vi "formatMsgDetails.vi"(8 "error in (no error)":errorcluster, 10 "msgCluster":T1={"msgName"="move", "msgDetails"=""}, 11 "TcpServerBase in":refnum<class "TcpServerBase.lvclass">) -> (0 "error out":errorcluster, 2 "jsonString":string, 3 "TcpServerBase out":refnum<class "TcpServerBase.lvclass">)   [LabVIEW 2018, in "TcpServerBase.lvclass"]
doc: "Convert the event or the telemetry message into a JSON format. If the message name has an empty string, an error will be created to inform other processes about this error."
uses:
  TcpServerBase.lvclass
  typedef/msgTypeDef.ctl
  <vilib>/Utility/error.llb/Error Cluster From Error Code.vi
  <vilib>/ErrorRing/Error Ring.xnode
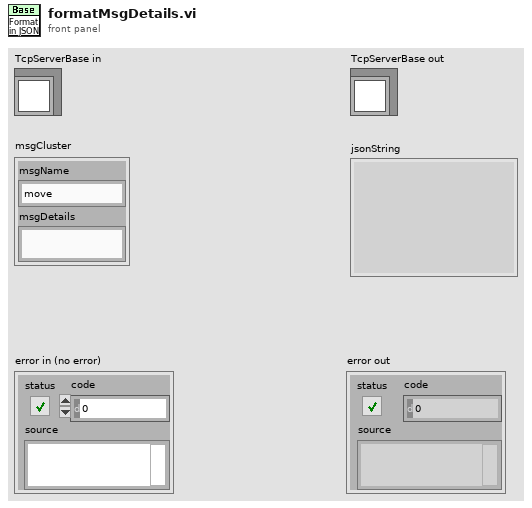
[diagram p1: front panel]
types:
  T1 = typedef "TcpServerBase.lvclass/msgTypeDef.ctl" = cluster{"msgName":string, "msgDetails":string}
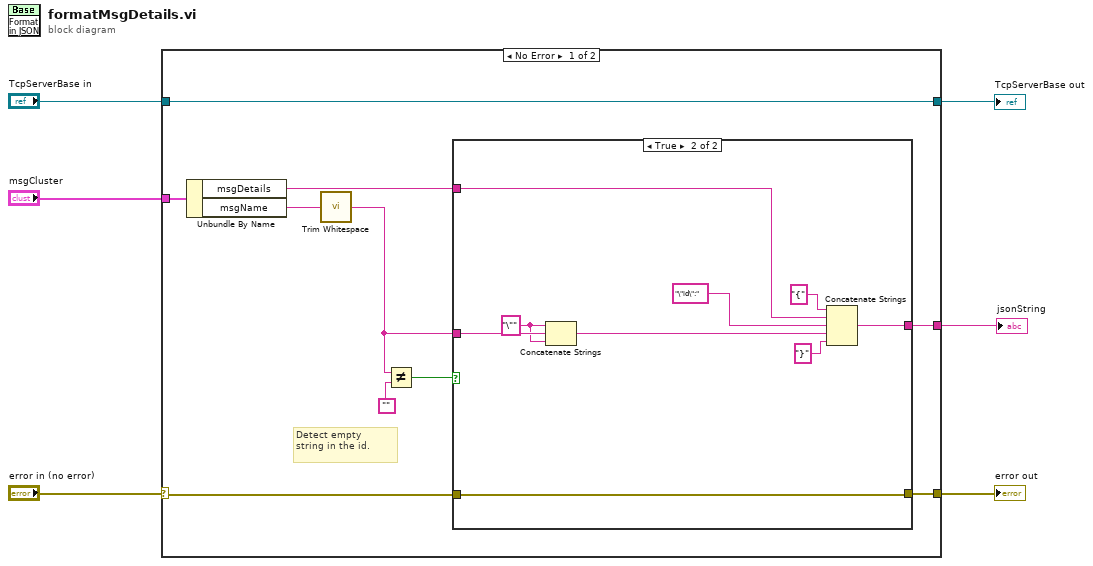
[diagram p0: block diagram]
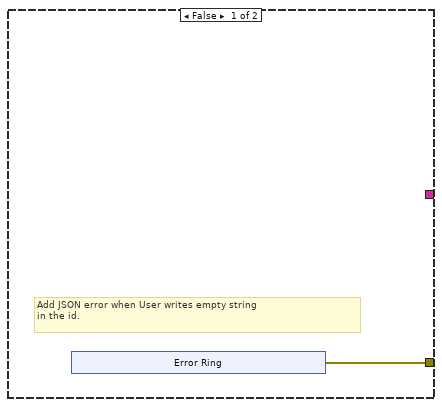
[diagram p2: hidden frame]
diagram:
  n1 = case shown="No Error" "error in (no error)" {
    selector: "error in (no error)" -> [w12 w31]
    tunnel: [w16 _] -> w2
    tunnel: "TcpServerBase in" -> [w15 w32]
    tunnel: [w15 w32] -> w4
    tunnel: [w11 w31] -> w3
    tunnel: "msgCluster" -> [w9 _]
    frame No Error {
      # "Detect empty\nstring in the id."
      n2 = Unbundle By Name(w9) -> ("msgDetails"=w7:string, "msgName"=w8:string)
      n3 = call <vilib>:"Trim Whitespace.vi"("string"=w8) -> ("trimmed string"=w10:string)  [unwired: 1 in]
      n4 = Not Equal?(x=w10, y="") -> (x != y?=w13:bool)
      n5 = case shown="True" w13 {
        tunnel: [_ w30] -> w16
        tunnel: w7 -> [_ w24]
        tunnel: w10 -> [_ w29]
        tunnel: w12 -> [_ w25]
        tunnel: [w17 w25] -> w11
        frame False {
          # "Add JSON error when User writes empty string\nin the id."
          n6 = xnode "Error Ring"() -> ("error out"=w17:errorcluster)
        }
        frame True {
          w26 = "\"" ("string")
          n7 = Concatenate Strings(w26, w29, w26) -> (w23:string)
          n8 = Concatenate Strings("{" ("string"), w24, "\"id\":", w23, "}" ("string")) -> (w30:string)
        }
      }
    }
    frame Error {
    }
  }
  "jsonString" <- w2
  "error out" <- w3
  "TcpServerBase out" <- w4
